vi "Sync Project.vi"() -> ()   [LabVIEW 2011, in "LVH-Toolbox.lvlib" / "LVH-Build-Tools.lvlib"]
doc: "This VI duplicates the install directories folder hierarchy in the source directory (if neccissary) and creates hard links in the source directory for each new file in the install directory. This VI should be run each time after LabVIEW development, before checking in code."
uses:
  LVH-Build-Tools.lvlib
  Private/Type Defs/Sync Source State.ctl
  System Tools/LVH-SystemTools.lvlib
panel:
  out "Error Out":errorcluster
  out "Window":enum32{"Init", "Configure", "Sync", "Summary"}(tab)
  in  "Config Help Button":bool
  in  "Settings Button":bool
  in  "Project":u16(ring) items=["LIFCK", "LVH-LINX"]
  in  "LabVIEW Version":u16(ring) items=["NI LabVIEW 2011 SP1"]
  in  "Config Next Button":bool
  in  "Config Cancel":bool
  out "Mass Compile Log":string
  out "Added Files":string[](array[string])
  in  "Summary Finish Button":bool
  out "Deleted Files":string[](array[string])
  out "Archive Link":string
  # "Sync Project\nInitializing..."
  # "Sync Project\n\nPlease choose a project to sync and the version of LabVIEW to sync from."
  # "Sync Project\n\nSyncing, please wait..."
  # "Sync Project\n\nSync complete.  Press Finish to exit."
  # "Backup Archive:"
  # "Mass Compile Log"
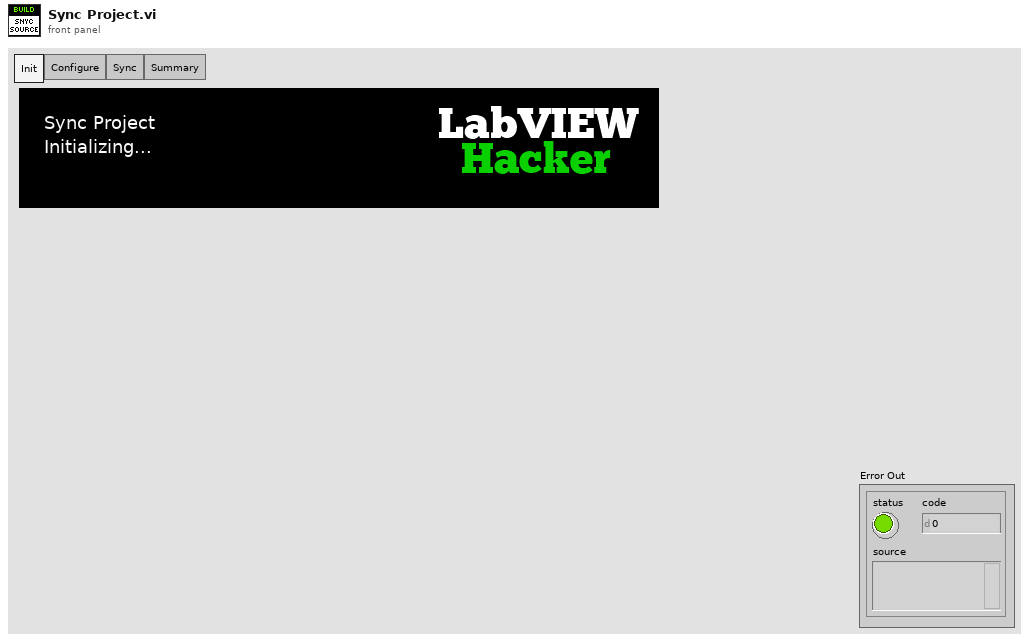
[diagram p1: front panel]
types:
  T1 = typedef "LVH-Toolbox.lvlib/LVH-Build-Tools.lvlib/Sync Source State.ctl" = enum16{"Init", "Configure", "Sync", "Summary"}
  T2 = typedef "LVH-Toolbox.lvlib/LVH-Build-Tools.lvlib/Sync Source Configuration.ctl" = cluster{"Installed Projects":T3[], "Project Source Root Dir":path, "All Config Files":path[], "Selected Project Config":path, "All LabVIEW Dirs":path[], "Selected LabVIEW Dir":path, "Backup Dir":path}
  T3 = typedef "LVH-Toolbox.lvlib/LVH-Build-Tools.lvlib/Installed Project.ctl" = cluster{"Project Name":string, "LV Versions":T4[], "Project Config Path":path}
  T4 = typedef "LVH-Toolbox.lvlib/LVH-SystemTools.lvlib/Installed LabVIEW Version.ctl" = cluster{"Version":string, "Path":path}
  T5 = typedef "LVH-Toolbox.lvlib/LVH-Build-Tools.lvlib/Configuration.ctl" = cluster{"Source Root":path, "Install Root":string, "Components":string[], "Ignore":string[], "Config Files":path[], "LV Directories":path[], "Install Paths":T6}
  T6 = typedef "LVH-Toolbox.lvlib/LVH-Build-Tools.lvlib/Install Configuration.ctl" = cluster{"LabVIEW Directory":path, "Project Source Config":path}
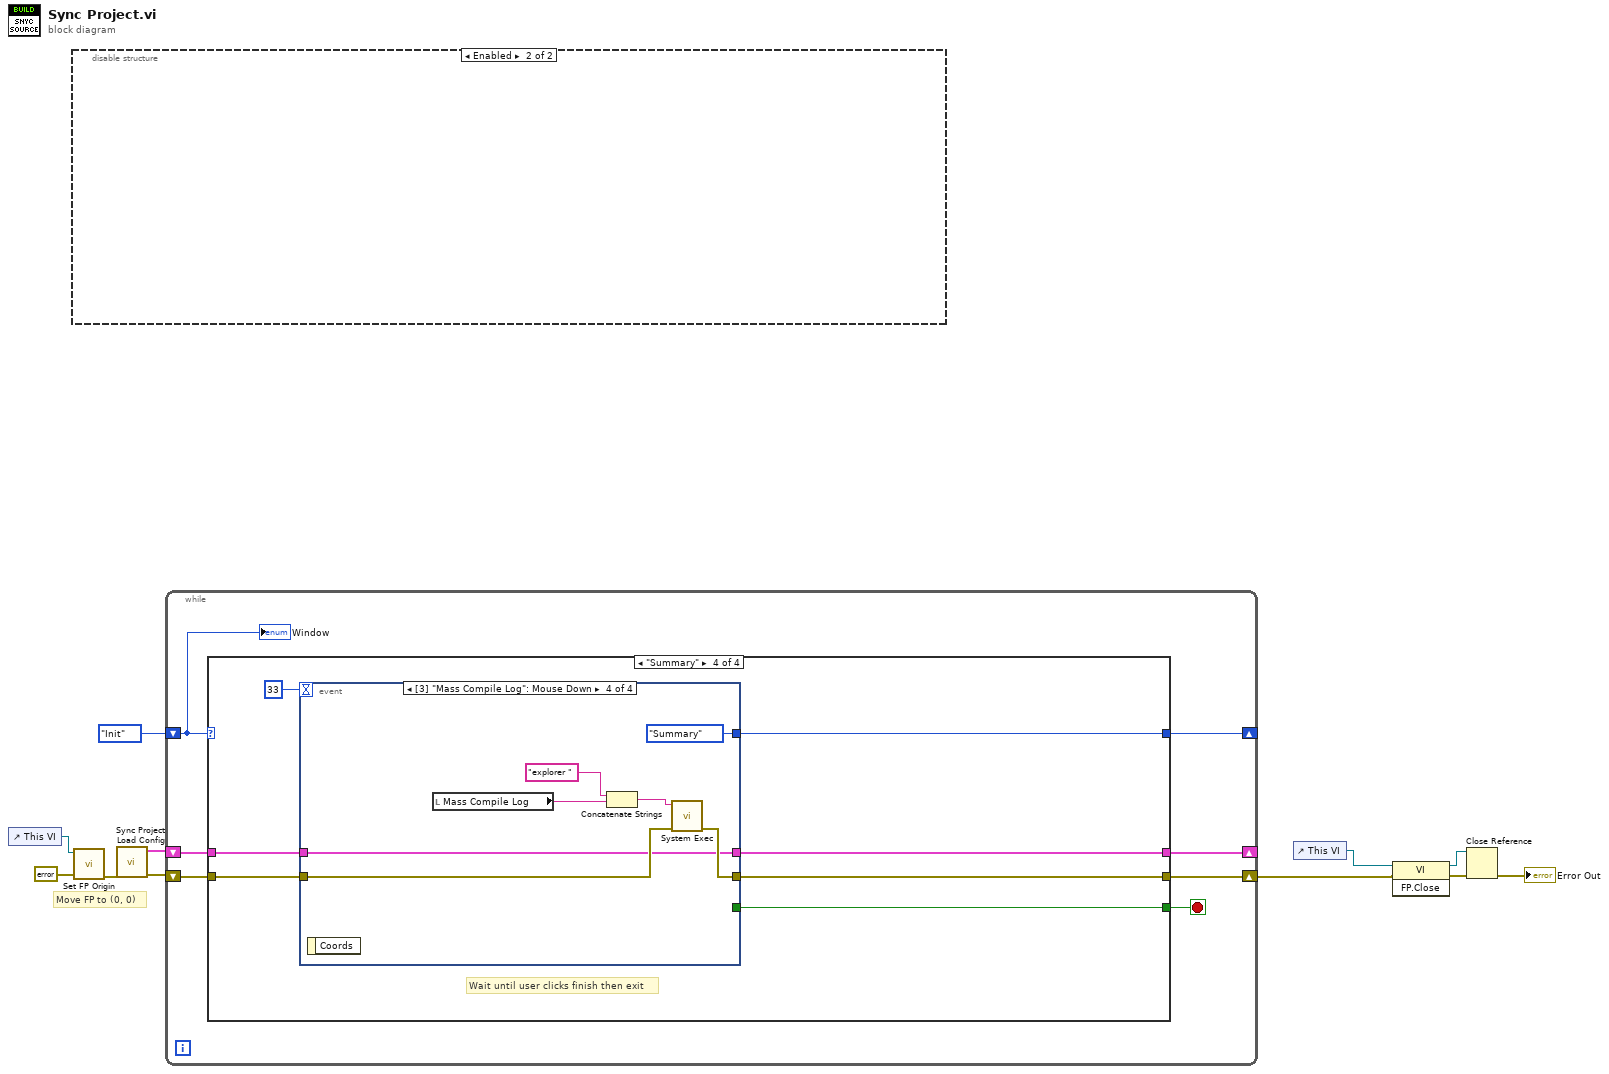
[diagram p0: block diagram]
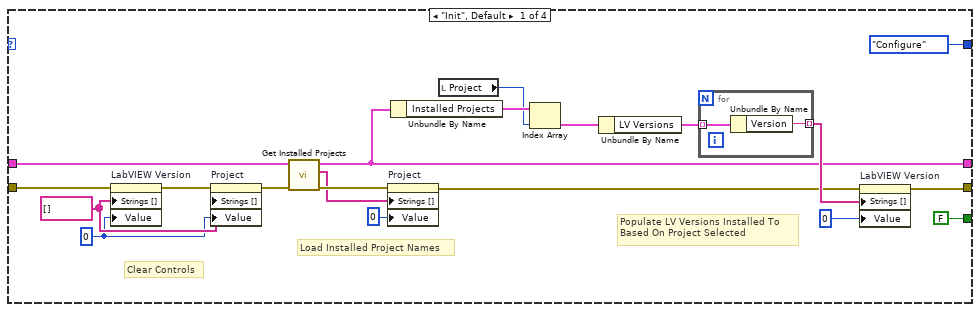
[diagram p2: hidden frame]
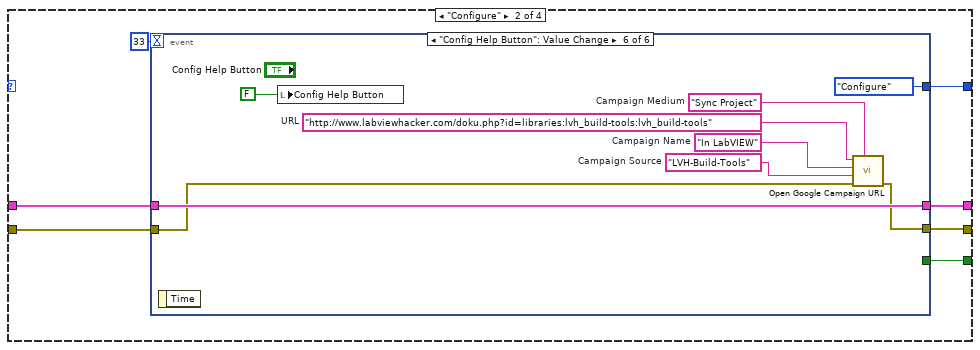
[diagram p3: hidden frame]
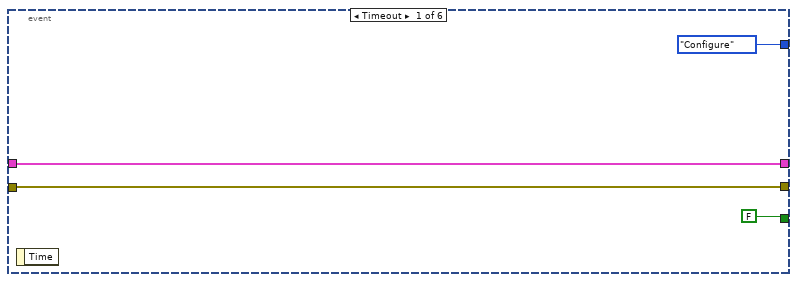
[diagram p4: hidden frame]
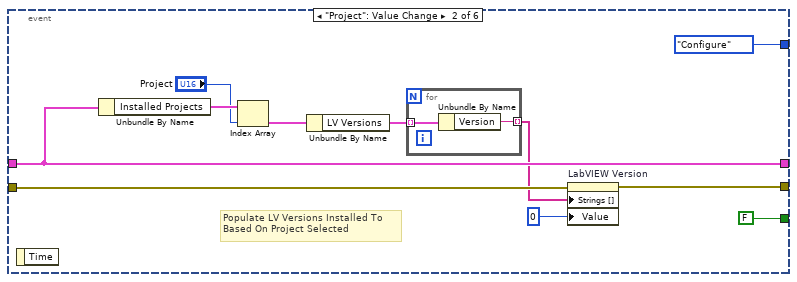
[diagram p5: hidden frame]
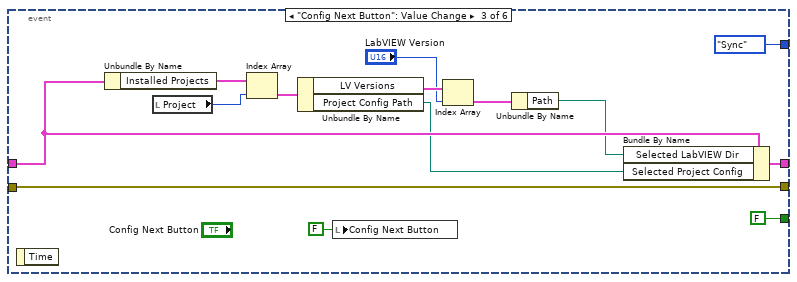
[diagram p6: hidden frame]
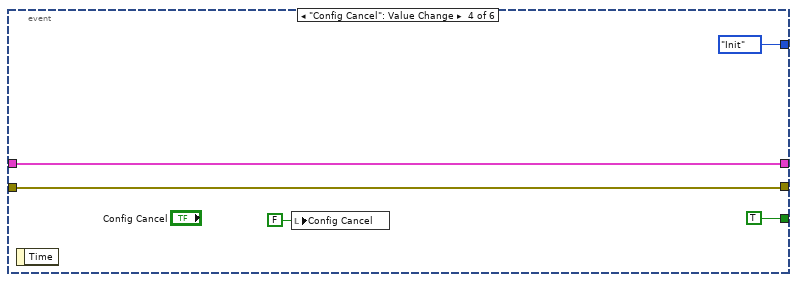
[diagram p7: hidden frame]
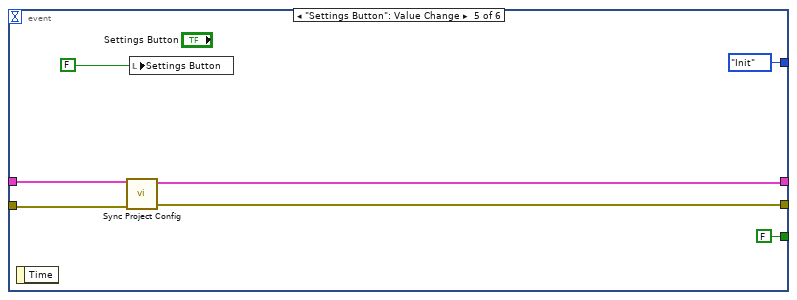
[diagram p8: hidden frame]
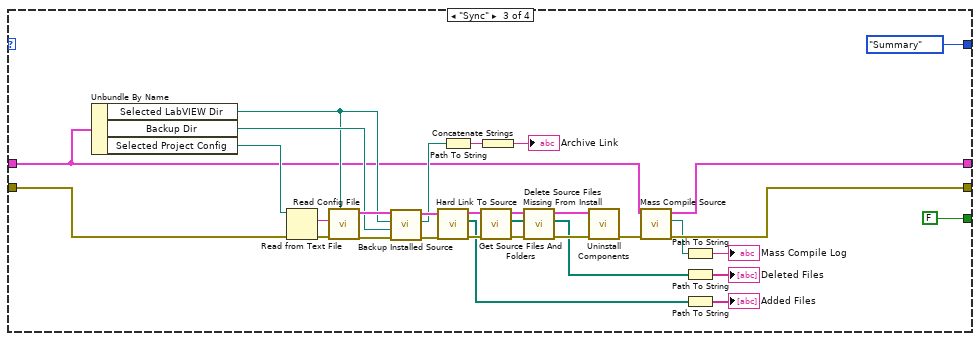
[diagram p9: hidden frame]
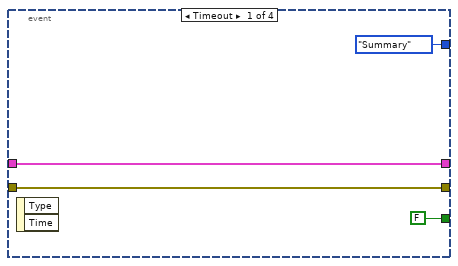
[diagram p10: hidden frame]
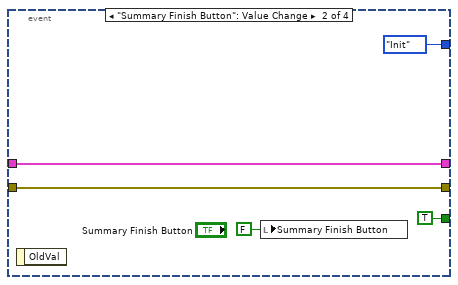
[diagram p11: hidden frame]
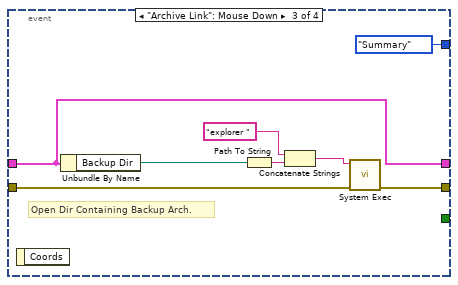
[diagram p12: hidden frame]
diagram:
  # "Move FP to (0, 0)"
  n1 = control-ref of="This VI"() -> (w10:refnum<vi>)
  n2 = disable-structure shown="Enabled" {
    frame Disabled {
    }
    frame Enabled {
    }
  }
  n3 = call "Set FP Origin.vi"("Error In"=errorcluster {"status"=FALSE, "code"=0, "source"=""} ("Error Out"), "VI Ref"=w10) -> ("Error Out"=w9:errorcluster)  [unwired: 9 in]
  n4 = call "Sync Project Load Config.vi"("Error In"=w9) -> ("Error Out"=w7:errorcluster, "Sync Source Config"=w8:T2)  [unwired: 7 in, 2 out]
  n5 = while {
    shift-right: [w13] -> _
    shift-left: Sync_Source_State."Init" ("Sync Source State") -> [w18]
    shift-right: [w15] -> w1
    shift-left: w7 -> [w17]
    shift-right: [w12] -> _
    shift-left: w8 -> [w16]
    stop <- w14 stop-if-true
    n6 = case shown="\"Summary\"" w18 {
      tunnel: w17 -> [w20 w46 w115 w138]
      tunnel: w16 -> [w19 w44 w103 w133]
      tunnel: [w25 w43 w114 w137] -> w15
      tunnel: [FALSE w45 FALSE w135] -> w14
      tunnel: [Sync_Source_State."Configure" ("Sync Source State") w41 Sync_Source_State."Summary" ("Sync Source State") w132] -> w13
      tunnel: [w27 w42 w102 w134] -> w12
      frame "Init", Default {
        w22 = u16 0
        w23 = string[] [] ("Strings []")
        # "Clear Controls"
        # "Populate LV Versions Installed To \nBased On Project Selected"
        # "Load Installed Project Names"
        n7 = property on="LabVIEW Version" class="Ring (strict)"(error in=w20, "Strings []"=w23, "Value"=w22) -> (error out=w24:errorcluster)  [unwired: 1 in, 1 out]
        n8 = property on="Project" class="Ring (strict)"(error in=w24, "Strings []"=w23, "Value"=w22) -> (error out=w21:errorcluster)  [unwired: 1 in, 1 out]
        n9 = call "Get Installed Projects.vi"("Error In"=w21, "Sync Source Config"=w19) -> ("Error Out"=w36:errorcluster, "Installed Projects"=w35:string[], "Sync Source Config"=w27:T2)  [unwired: 7 in]
        n10 = property on="Project" class="Ring (strict)"(error in=w36, "Strings []"=w35, "Value"=u16 0) -> (error out=w26:errorcluster)  [unwired: 1 in, 1 out]
        n11 = Unbundle By Name(w27) -> ("Installed Projects"=w33:T3[])
        n12 = local read "Project"() -> (w28:u16)
        n13 = Index Array(array=w33, index=w28) -> (element=w32:T3)
        n14 = Unbundle By Name(w32) -> ("LV Versions"=w31:T4[])
        n15 = for {
          tunnel: w31 -> [w40] mode=indexing
          tunnel: [w39] -> w30 mode=indexing
          n16 = Unbundle By Name(w40) -> ("Version"=w39:string)
        }
        n17 = property on="LabVIEW Version" class="Ring (strict)"(error in=w26, "Strings []"=w30, "Value"=u16 0) -> (error out=w25:errorcluster)  [unwired: 1 in, 1 out]
      }
      frame "Configure" {
        n18 = event shown="[5] \"Config Help Button\": Value Change" {
          selector: _ -> [_ _ _ _ _ _]
          dyn-events: _ -> [_ _ _ _ _ _]
          timeout: 33 ("Numeric Control") -> [_ _ _ _ _ _]
          tunnel: w46 -> [w49 w60 w68 w81 w89 w97]
          tunnel: [FALSE FALSE FALSE TRUE FALSE _] -> w45
          tunnel: w44 -> [w50 w56 w74 w80 w88 w99]
          tunnel: [w49 w57 w68 w81 w86 w96] -> w43
          tunnel: [w50 w56 w69 w80 w87 w99] -> w42
          tunnel: [Sync_Source_State."Configure" ("Sync Source State") Sync_Source_State."Configure" ("Sync Source State") Sync_Source_State."Sync" ("Sync Source State") Sync_Source_State."Init" ("Sync Source State") Sync_Source_State."Init" ("Sync Source State") Sync_Source_State."Configure" ("Sync Source State")] -> w41
          event Timeout {
            n19 = event-data() -> ()  [unwired: 1 in, 1 out]
          }
          event "Project": Value Change {
            # "Populate LV Versions Installed To \nBased On Project Selected"
            n20 = event-data() -> ()  [unwired: 1 in, 1 out]
            n21 = Unbundle By Name(w56) -> ("Installed Projects"=w62:T3[])
            n22 = Index Array(array=w62, index="Project") -> (element=w59:T3)
            n23 = Unbundle By Name(w59) -> ("LV Versions"=w55:T4[])
            n24 = for {
              tunnel: w55 -> [w64] mode=indexing
              tunnel: [w63] -> w54 mode=indexing
              n25 = Unbundle By Name(w64) -> ("Version"=w63:string)
            }
            n26 = property on="LabVIEW Version" class="Ring (strict)"(error in=w60, "Strings []"=w54, "Value"=u16 0) -> (error out=w57:errorcluster)  [unwired: 1 in, 1 out]
          }
          event "Config Next Button": Value Change {
            n27 = event-data() -> ()  [unwired: 1 in, 1 out]
            n28 = Unbundle By Name(w74) -> ("Installed Projects"=w77:T3[])
            n29 = local read "Project"() -> (w76:u16)
            n30 = Index Array(array=w77, index=w76) -> (element=w75:T3)
            n31 = Unbundle By Name(w75) -> ("LV Versions"=w73:T4[], "Project Config Path"=w70:path)
            n32 = local write "Config Next Button"(FALSE ("Config Next Button")) -> ()
            n33 = Index Array(array=w73, index="LabVIEW Version") -> (element=w71:T4)
            n34 = Unbundle By Name(w71) -> ("Path"=w65:path)
            n35 = Bundle By Name(cluster=w74, "Selected LabVIEW Dir"=w65, "Selected Project Config"=w70) -> (w69:T2)
          }
          event "Config Cancel": Value Change {
            n36 = event-data() -> ()  [unwired: 1 in, 1 out]
            n37 = local write "Config Cancel"(FALSE ("Config Cancel")) -> ()
          }
          event "Settings Button": Value Change {
            n38 = event-data() -> ()  [unwired: 1 in, 1 out]
            n39 = call "Sync Project Config.vi"("Error In"=w89, "Sync Source Config"=w88) -> ("Error Out"=w86:errorcluster, "Sync Source Config"=w87:T2)  [unwired: 8 in]
            n40 = local write "Settings Button"(FALSE ("Settings Button")) -> ()
          }
          event "Config Help Button": Value Change {
            w92 = "LVH-Build-Tools"  # Campaign Source
            w93 = "In LabVIEW"  # Campaign Name
            w94 = "Sync Project"  # Campaign Medium
            w95 = "http://www.labviewhacker.com/doku.php?id=libraries:lvh_build-tools:lvh_build-tools"  # URL
            n41 = event-data() -> ()  [unwired: 1 in, 1 out]
            n42 = local write "Config Help Button"(FALSE ("Help Button")) -> ()
            n43 = call "Open Google Campaign URL.vi"("Campaign Medium"=w94, "Error In"=w97, "Campaign Source"=w92, "Campaign Name"=w93, "URL"=w95) -> ("Error Out"=w96:errorcluster)  [unwired: 5 in, 1 out]
          }
        }
      }
      frame "Sync" {
        n44 = Unbundle By Name(w103) -> ("Selected LabVIEW Dir"=w104:path, "Backup Dir"=w106:path, "Selected Project Config"=w105:path)
        n45 = Read from Text File(file (use dialog)=w105, error in=w115) -> (text=w117:string, error out=w116:errorcluster)  [unwired: 2 in, 2 out]
        n46 = call "Read Config File.vi"("LabVIEW Dir Override"=w104, "error in (no error)"=w116, "Config File In"=w117) -> ("error out"=w126:errorcluster, "Configuration out"=w125:T5)  [unwired: 7 in]
        n47 = call "Backup Installed Source.vi"("Error In"=w126, "Backup Dir"=w106, "LabVIEW Dir"=w104, "Configuration"=w125) -> ("Error Out"=w127:errorcluster, "Archive Dest"=w107:path, "Configuration"=w128:T5)  [unwired: 5 in]
        n48 = call "Hard Link To Source.vi"("Error In"=w127, "Configuration in"=w128) -> ("Error Out"=w118:errorcluster, "Files Added To Source"=w111:path[], "Configuration out"=w122:T5)  [unwired: 7 in]
        n49 = Path To String(path=w107) -> (string=w109:string)
        n50 = call "Get Source Files And Folders.vi"("Error In"=w118, "Configuration"=w122) -> ("Error Out"=w119:errorcluster, "All Source Files"=w121:path[], "Configuration"=w120:T5)  [unwired: 6 in, 1 out]
        n51 = Concatenate Strings(w109) -> (→"Archive Link":string)
        n52 = call "Delete Source Files Missing From Install.vi"("Error In"=w119, "Source Files"=w121, "Configuration"=w120) -> ("Error Out"=w123:errorcluster, "Deleted From Souce"=w113:path[], "Configuration"=w124:T5)  [unwired: 6 in]
        n53 = call "Uninstall Components.vi"("error in (no error)"=w123, "Configuration in"=w124) -> ("error out"=w129:errorcluster)  [unwired: 7 in, 2 out]
        n54 = call "Mass Compile Source.vi"("Error In"=w129, "Sync Source Config"=w103) -> ("Error Out"=w114:errorcluster, "Mass Compile Log"=w100:path, "Sync Source Config"=w102:T2)  [unwired: 7 in]
        n55 = Path To String(path=w100) -> (string=→"Mass Compile Log":string)
        n56 = Path To String(path=w113) -> (string=→"Deleted Files":string[])
        n57 = Path To String(path=w111) -> (string=→"Added Files":string[])
      }
      frame "Summary" {
        # "Wait until user clicks finish then exit"
        n58 = event shown="[3] \"Mass Compile Log\": Mouse Down" {
          selector: _ -> [_ _ _ _]
          dyn-events: _ -> [_ _ _ _]
          timeout: 33 -> [_ _ _ _]
          tunnel: w138 -> [w142 w146 w151 w158]
          tunnel: [w142 w146 w152 w160] -> w137
          tunnel: [FALSE TRUE _ _] -> w135
          tunnel: [w140 w144 w148 w157] -> w134
          tunnel: w133 -> [w140 w144 w148 w157]
          tunnel: [Sync_Source_State."Summary" ("Sync Source State") Sync_Source_State."Init" ("Sync Source State") Sync_Source_State."Summary" ("Sync Source State") Sync_Source_State."Summary" ("Sync Source State")] -> w132
          event Timeout {
            n59 = event-data() -> ()  [unwired: 1 in, 2 out]
          }
          event "Summary Finish Button": Value Change {
            n60 = event-data() -> ()  [unwired: 1 in, 1 out]
            n61 = local write "Summary Finish Button"(FALSE ("Summary Finish Button")) -> ()
          }
          event "Archive Link": Mouse Down {
            # "Open Dir Containing Backup Arch."
            n62 = event-data() -> ()  [unwired: 1 in, 1 out]
            n63 = Unbundle By Name(w148) -> ("Backup Dir"=w149:path)
            n64 = Path To String(path=w149) -> (string=w154:string)
            n65 = Concatenate Strings("explorer " ("string"), w154) -> (w153:string)
            n66 = call <vilib>:"System Exec.vi"("error in (no error)"=w151, "command line"=w153) -> ("error out"=w152:errorcluster)  [unwired: 6 in, 3 out]
          }
          event "Mass Compile Log": Mouse Down {
            n67 = event-data() -> ()  [unwired: 1 in, 1 out]
            n68 = local read "Mass Compile Log"() -> (w159:string)
            n69 = Concatenate Strings("explorer " ("string"), w159) -> (w161:string)
            n70 = call <vilib>:"System Exec.vi"("error in (no error)"=w158, "command line"=w161) -> ("error out"=w160:errorcluster)  [unwired: 6 in, 3 out]
          }
        }
      }
    }
    "Window" <- w18
  }
  n71 = control-ref of="This VI"() -> (w4:refnum<vi>)
  n72 = invoke class="VI" method="FP.Close"(reference=w4, error in=w1) -> (reference out=w3:refnum<vi>, error out=w2:errorcluster)  [unwired: 1 in, 1 out]
  n73 = Close Reference(reference=w3, error in (no error)=w2) -> (error out=→"Error Out":errorcluster)
